vi "ReadINIScript.vi"(8 "error in (no error)":errorcluster, 10 "Script Name":string, 11 "INI File Path":path) -> (0 "error out":errorcluster, 1 "Script with $":string[](array[string]), 2 "found?":bool, 3 "Script":string[](array[string]))   [LabVIEW 2018, in "Test.lvclass"]
uses:
  Test.lvclass
  <vilib>/Utility/config.llb/NI_LVConfig.lvlib
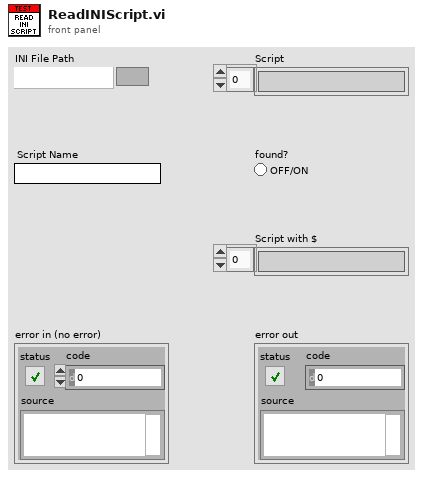
[diagram p1: front panel]
types:
  T1 = typedef "NI_LVConfig.lvlib/Config Data RefNum.ctl" = refnum<k1>
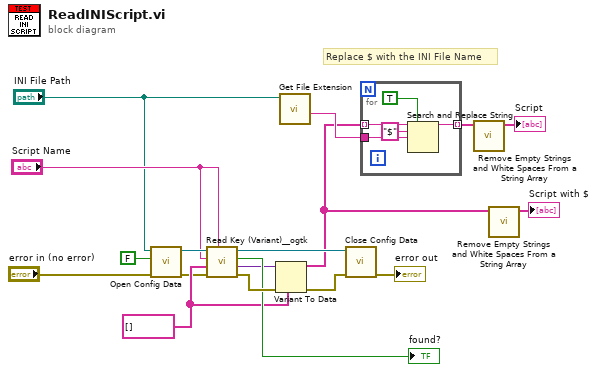
[diagram p0: block diagram]
diagram:
  w12 = string[] []
  # "Replace $ with the INI File Name"
  n1 = call <vilib>:"Open Config Data.vi"("error in (no error)"="error in (no error)", "create file if necessary (T)"=FALSE, "configuration file path"="INI File Path") -> ("error out"=w10:errorcluster, "refnum"=w9:T1)  [unwired: 6 in, 1 out]
  n2 = call <userlib>:"Read Key (Variant)__ogtk.vi"("section"="Script Name", "error in (no error)"=w10, "type"=w12, "key (optional)"="Script Name", "refnum"=w9) -> ("error out"=w18:errorcluster, "key-value"=w11:variant, "found?"=→"found?":bool, "refnum out"=w14:T1)  [unwired: 3 in]
  n3 = Variant To Data(error in=w18, type=w12, Variant=w11) -> (data=w2:string[], error out=w15:errorcluster)
  n4 = call <vilib>:"Get File Extension.vi"("file"="INI File Path") -> ("filename without extension"=w5:string)  [unwired: 6 in, 4 out]
  n5 = call <vilib>:"Close Config Data.vi"("error in (no error)"=w15, "refnum"=w14) -> ("error out"=→"error out":errorcluster)  [unwired: 8 in, 1 out]
  n6 = for {
    tunnel: w2 -> [w23] mode=indexing
    tunnel: w5 -> [w20]
    tunnel: [w19] -> w3 mode=indexing
    n7 = Search and Replace String(replace all?=TRUE ("replace all? (F)"), input string=w23, search string="$", replace string=w20) -> (result string=w19:string)  [unwired: 4 in, 3 out]
  }
  n8 = call "Remove Empty Strings and White Spaces From a String Array.vi"("Array in"=w3) -> ("Array out"=→"Script":string[])  [unwired: 10 in]
  n9 = call "Remove Empty Strings and White Spaces From a String Array.vi"("Array in"=w2) -> ("Array out"=→"Script with $":string[])  [unwired: 10 in]
